vi "getAxisLetter.vi"(8 "error in (no error)":errorcluster, 11 "Axis in":refnum<class "Axis.lvclass">) -> (0 "error out":errorcluster, 2 "Axis Letter":string, 3 "Axis out":refnum<class "Axis.lvclass">)   [LabVIEW 2019, in "Axis.lvclass"]
uses:
  Axis.lvclass
  Axis.lvclass/Axis.ctl
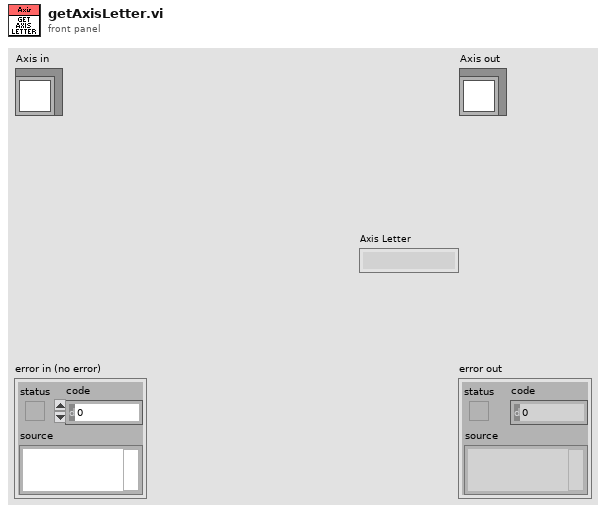
[diagram p1: front panel]
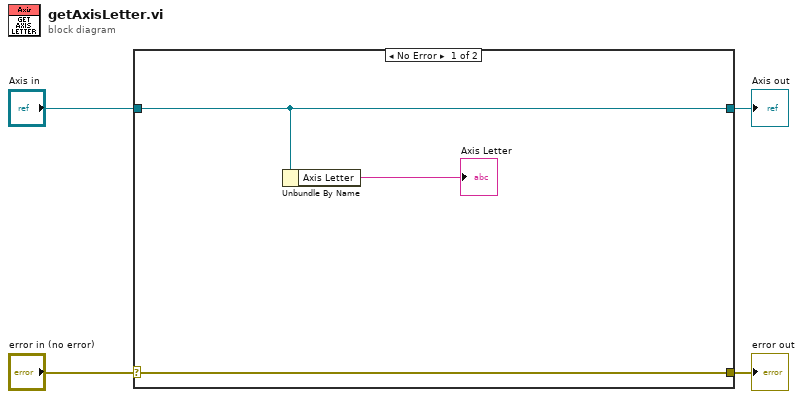
[diagram p0: block diagram]
diagram:
  n1 = case shown="No Error" "error in (no error)" {
    selector: "error in (no error)" -> [w7 w9]
    tunnel: [w7 w9] -> w3
    tunnel: [w5 w8] -> w1
    tunnel: "Axis in" -> [w5 w8]
    frame No Error {
      n2 = Unbundle By Name(w5) -> ("Axis Letter"=→"Axis Letter":string)
    }
    frame Error {
    }
  }
  "error out" <- w3
  "Axis out" <- w1
